vi "WBRGB_separate_sub.vi"(5 "WB_RGB":dbl[][](array[numeric])) -> (0 "WB_B":dbl[][](array[numeric]), 1 "WB_G":dbl[][](array[numeric]), 2 "WB_R":dbl[][](array[numeric]))   [LabVIEW 2021]
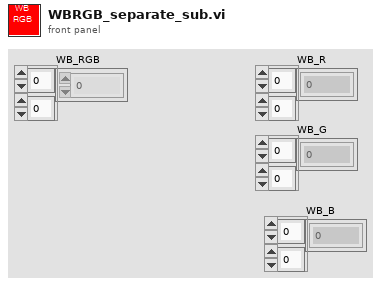
[diagram p1: front panel]
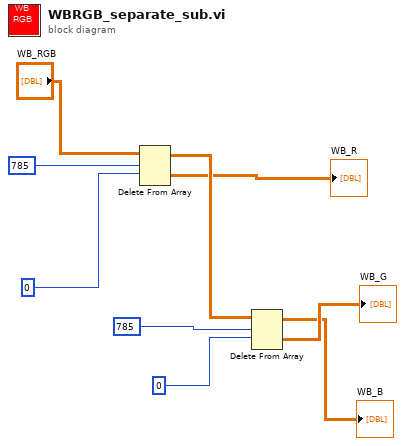
[diagram p0: block diagram]
diagram:
  n1 = Delete From Array(array="WB_RGB", length=785 ("길이"), index (row)=0 ("인덱스")) -> (deleted portion=→"WB_R":dbl[][], array with subset deleted=w6:dbl[][])  [unwired: 1 in]
  n2 = Delete From Array(array=w6, length=785 ("길이"), index (row)=0 ("인덱스 (행)")) -> (deleted portion=→"WB_G":dbl[][], array with subset deleted=→"WB_B":dbl[][])  [unwired: 1 in]
